vi "Get Version Independent.vi"(8 "error in (no error)":errorcluster, 11 "NI_AB_API_Application in":refnum<class "NI_AB_API_Application.lvclass">) -> (0 "error out":errorcluster, 2 "versionIndependent":bool, 3 "NI_AB_API_Application out":refnum<class "NI_AB_API_Application.lvclass">)   [LabVIEW 2020, in "NI_AB_API_Application.lvclass"]
uses:
  <vilib>/AppBuilder/AB_API/Application/NI_AB_API_Application.lvclass
  <vilib>/AppBuilder/AB_API/Targetfile/NI_AB_API_Targetfile.lvclass
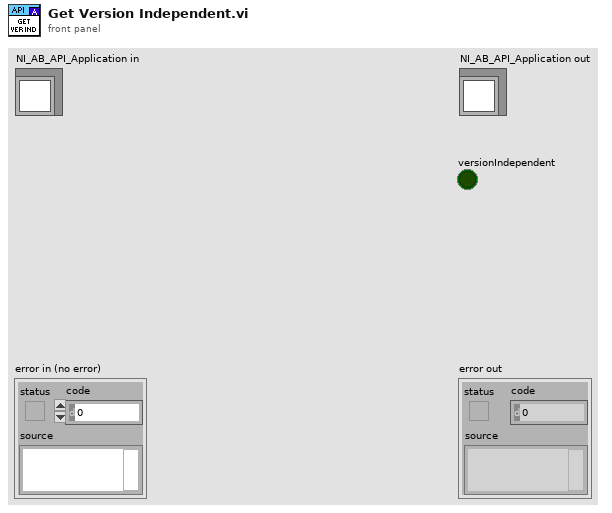
[diagram p1: front panel]
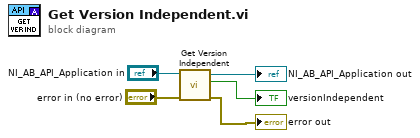
[diagram p0: block diagram]
diagram:
  n1 = call-parent "Get Version Independent.vi"("error in (no error)"="error in (no error)", "NI_AB_API_Targetfile in"="NI_AB_API_Application in") -> ("error out"=→"error out":errorcluster, "versionIndependent"=→"versionIndependent":bool, "NI_AB_API_Targetfile out"=→"NI_AB_API_Application out":refnum<class "NI_AB_API_Application.lvclass">)  [unwired: 7 in]
